vi "Property Node (Filesystem Statistics).vi"   [LabVIEW 2020, in "NI_SFTP.lvlib"]
doc: "Gets (reads) remote filesystem statistics returned by the <b>Get Filesystem Statistics</b> function."
uses:
  <vilib>/net/SFTP/NI_SFTP.lvlib
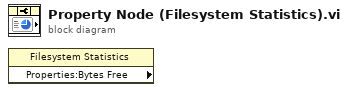
[diagram p0: block diagram]
diagram:
  n1 = property class="Filesystem Statistics" props=["Properties:Bytes Free"]() -> ()  [unwired: 2 in, 3 out]
